vi "DSCServVI.vi"() -> ()   [LabVIEW 2011]
panel:
  in  "SAM":dbl
  out "GERRY":dbl
  out "FRED":dbl
  in  "stop":bool
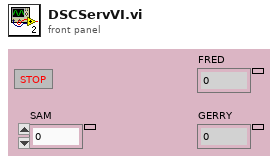
[diagram p1: front panel]
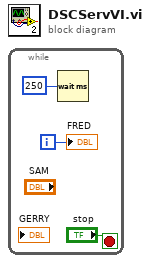
[diagram p0: block diagram]
diagram:
  n1 = while {
    i -> [w1]
    stop <- "stop" stop-if-true
    n2 = Wait (ms)(milliseconds to wait=u32 250) -> ()  [unwired: 1 out]
    "FRED" <- w1
  }
